vi "IonPumpPressure.vi"() -> ()   [LabVIEW 2010]
panel:
  in  "TC Switch":bool caption="AC Pressure"
  in  "AC Switch":bool caption="AC Pressure"
  out "TC Pressure (Torr)":dbl
  out "TC Pressure":cluster{dbl, dbl}[](graph)
  out "AC Pressure":cluster{dbl, dbl}[](graph)
  out "AC Pressure (Torr)":dbl
  # "ION PUMP CONTROLLER\nPRESSURE GAUGE"
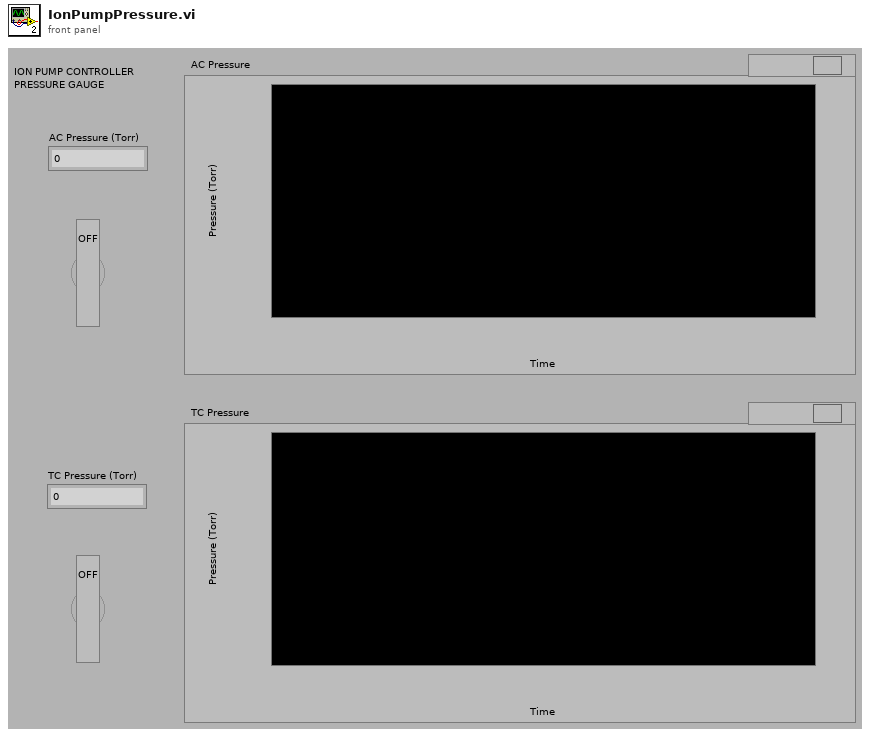
[diagram p1: front panel]
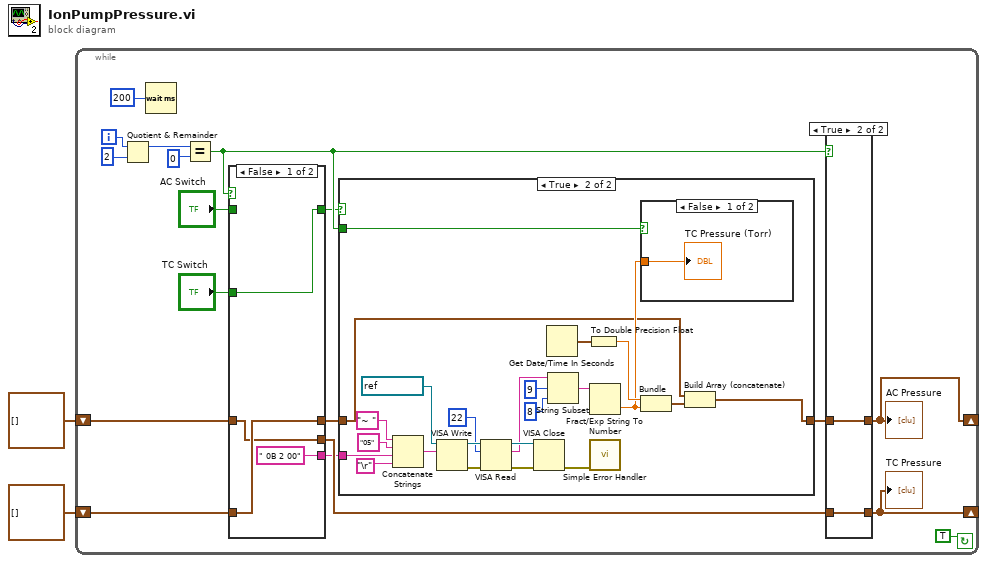
[diagram p0: block diagram]
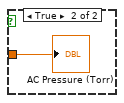
[diagram p3: hidden frame]
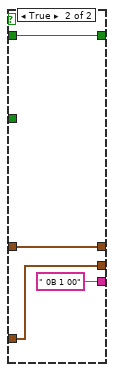
[diagram p4: hidden frame]
diagram:
  n1 = while {
    shift-right: [w8] -> _
    shift-left: cluster{dbl, dbl}[] [] -> [w17]
    shift-right: [w7] -> _
    shift-left: cluster{dbl, dbl}[] [] -> [w15]
    i -> [w13]
    stop <- TRUE continue-if-true
    n2 = Quotient & Remainder(x=w13, y=2) -> (x-y*floor(x/y)=w11:i32)  [unwired: 1 out]
    n3 = Wait (ms)(milliseconds to wait=u32 200) -> ()  [unwired: 1 out]
    n4 = Equal?(x=w11, y=0) -> (x = y?=w6:bool)
    n5 = case shown="False" w6 {
      tunnel: w17 -> [w49 w54]
      tunnel: [w50 w54] -> w16
      tunnel: w15 -> [w50 w53]
      tunnel: [w49 w53] -> w14
      tunnel: [" 0B 2 00" ("string") " 0B 1 00" ("string")] -> w9
      tunnel: "AC Switch" -> [_ w51]
      tunnel: [w47 w51] -> w5
      tunnel: "TC Switch" -> [w47 _]
      frame False {
      }
      frame True {
      }
    }
    n6 = case shown="True" w5 {
      tunnel: [w21 w25] -> w18
      tunnel: w16 -> [w21 w24]
      tunnel: w9 -> [_ w23]
      tunnel: w6 -> [_ w22]
      frame False {
      }
      frame True {
        n7 = Concatenate Strings("~ " ("string"), "05" ("string"), w23, "\r") -> (w44:string)
        n8 = VISA Write(VISA resource name=refnum<visa-resource-name> "COM3", write buffer=w44) -> (VISA resource name out=w42:refnum<visa-resource-name>, error out=w38:errorcluster)  [unwired: 1 in, 1 out]
        n9 = VISA Read(VISA resource name=w42, byte count=u32 22, error in (no error)=w38) -> (VISA resource name out=w41:refnum<visa-resource-name>, read buffer=w33:string, error out=w39:errorcluster)  [unwired: 1 out]
        n10 = VISA Close(VISA resource name=w41, error in (no error)=w39) -> (error out=w40:errorcluster)
        n11 = Get Date/Time In Seconds() -> (seconds since 1Jan1904=w29:timestamp)
        n12 = String Subset(string=w33, offset (0)=9, length (rest)=8 ("length (rest)")) -> (substring=w30:string)
        n13 = To Double Precision Float(number=w29) -> (double precision float=w28:dbl)
        n14 = Fract/Exp String To Number(string=w30) -> (number=w27:dbl)  [unwired: 3 in, 1 out]
        n15 = call <vilib>:"Simple Error Handler.vi"("error in (no error)"=w40) -> ()  [unwired: 4 in, 5 out]
        n16 = case shown="False" w22 {
          tunnel: w27 -> [w45 w46]
          frame False {
            "TC Pressure (Torr)" <- w45
          }
          frame True {
            "AC Pressure (Torr)" <- w46
          }
        }
        n17 = Bundle(w28, w27) -> (w26:cluster{dbl, dbl})  [unwired: 1 in]
        n18 = Build Array (concatenate)(w24, w26) -> (w25:cluster{dbl, dbl}[])
      }
    }
    n19 = case shown="True" w6 {
      tunnel: w18 -> [w56 w58]
      tunnel: [w55 w58] -> w8
      tunnel: [w56 w57] -> w7
      tunnel: w14 -> [w55 w57]
      frame False {
      }
      frame True {
      }
    }
    "AC Pressure" <- w8
    "TC Pressure" <- w7
  }
